vi "G_beepalert.vi"() -> ()   [LabVIEW 2015]
panel:
  in  "frequency (Hz)":u32=1200
  in  "duration (msec)":u32=100
  out "beep":bool
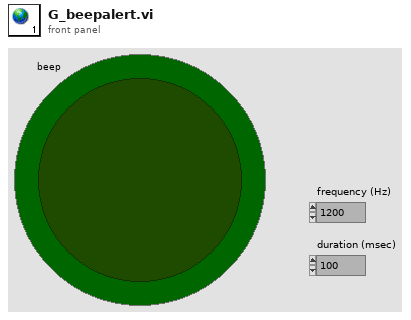
[diagram p1: front panel]
diagram:
